vi "Send Request (Sync).vi"(6 "Timeout (-1)":i32=-1, 8 "error in (no error)":errorcluster, 10 "JSON Request String":string, 11 "JSONRPC Server in":refnum<class "JSONRPC Server.lvclass">) -> (0 "error out":errorcluster, 2 "JSON Response String":string, 3 "JSONRPC Server out":refnum<class "JSONRPC Server.lvclass">)   [LabVIEW 2016, in "JSONRPC Server.lvclass"]
uses:
  JSONRPC Server.lvclass
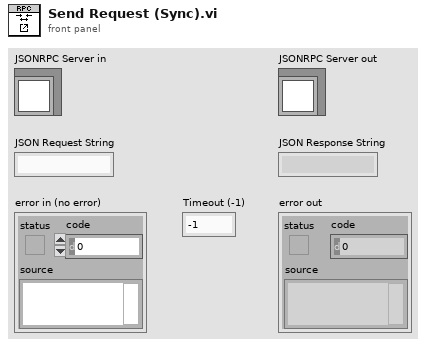
[diagram p1: front panel]
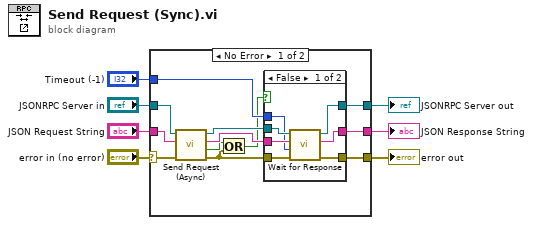
[diagram p0: block diagram]
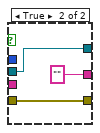
[diagram p2: hidden frame]
diagram:
  n1 = case shown="No Error" "error in (no error)" {
    selector: "error in (no error)" -> [w13 w31]
    tunnel: [w12 w31] -> w6
    tunnel: [w17 w30] -> w4
    tunnel: "JSONRPC Server in" -> [w18 w30]
    tunnel: "JSON Request String" -> [w15 _]
    tunnel: [w14 _] -> w2
    tunnel: "Timeout (-1)" -> [w11 _]
    frame No Error {
      n2 = call "Send Request (Async).vi"("error in (no error)"=w13, "JSON Request String"=w15, "Server in"=w18) -> ("error out"=w9:errorcluster, "notification?"=w10:bool, "id value"=w16:string, "Server out"=w19:refnum<class "JSONRPC Server.lvclass">)  [unwired: 5 in]
      n3 = Or(x=w10, y=w9) -> (x .or. y?=w8:bool)
      n4 = case shown="False" w8 {
        tunnel: w19 -> [w26 w29]
        tunnel: [w25 w29] -> w17
        tunnel: w16 -> [w24 _]
        tunnel: w9 -> [w23 w28]
        tunnel: [w22 "" ("JSON Response String")] -> w14
        tunnel: [w21 w28] -> w12
        tunnel: w11 -> [w20 _]
        frame False {
          n5 = call-dynamic "Wait for Response.vi"("error in (no error)"=w23, "Timeout (-1)"=w20, "id String"=w24, "JSONRPC Server in"=w26) -> ("error out"=w21:errorcluster, "JSON Response String"=w22:string, "JSONRPC Server out"=w25:refnum<class "JSONRPC Server.lvclass">)  [unwired: 5 in]
        }
        frame True {
        }
      }
    }
    frame Error {
    }
  }
  "error out" <- w6
  "JSONRPC Server out" <- w4
  "JSON Response String" <- w2
